vi "Main.vi"() -> ()   [LabVIEW 2009, in "Main.lvlib"]
doc: "Main robot program VI. Should be the start VI of the built program."
uses:
  Main.lvlib
  Drive/Drive_Point.ctl
  OWNCAN.lvlib
  NetworkVarTarget.lvlib
  MainVariables.lvlib
  Drive.lvlib
panel:
  in  "Goal point":T1
  out "error out":errorcluster
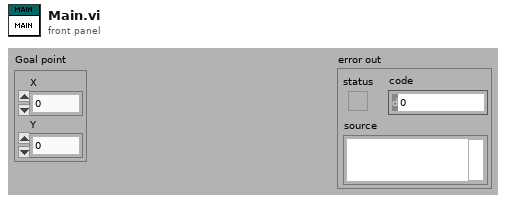
[diagram p1: front panel]
types:
  T1 = typedef "Drive.lvlib/Drive_Point.ctl" = cluster{"X":dbl, "Y":dbl}
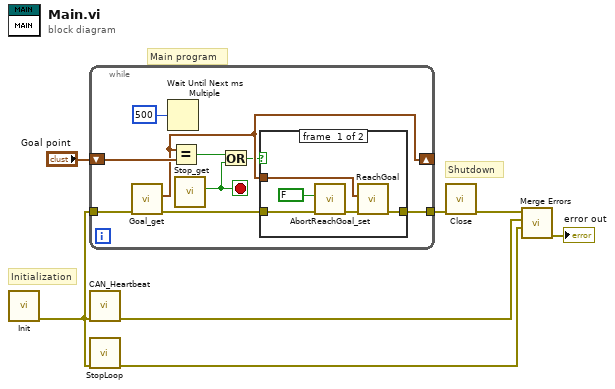
[diagram p0: block diagram]
diagram:
  # "Shutdown"
  # "Main program"
  # "Initialization"
  n1 = call "Init.vi"() -> ("error out"=w1:errorcluster)  [unwired: 11 in]
  n2 = while {
    tunnel: [w16] -> w7
    tunnel: w1 -> [w14]
    shift-right: [w11] -> _
    shift-left: "Goal point" -> [w15]
    stop <- w9 stop-if-true
    n3 = call "Goal_get.vi"("error in (no error)"=w14) -> ("error out"=w13:errorcluster, "Goal"=w11:cluster{"X":dbl, "Y":dbl})  [unwired: 9 in]
    n4 = Wait Until Next ms Multiple(millisecond multiple=u32 500) -> ()  [unwired: 1 out]
    n5 = Equal?(x=w11, y=w15) -> (x = y?=w8:bool)
    n6 = call "Stop_get.vi"() -> ("Stop"=w9:bool)  [unwired: 10 in, 1 out]
    n7 = Or(x=w8, y=w9) -> (x .or. y?=w10:bool)
    n8 = case shown="False" w10 {
      tunnel: [w21 w22] -> w16
      tunnel: w13 -> [w19 w22]
      tunnel: w11 -> [w18 _]
      frame #0 {
        n9 = call "AbortReachGoal_set.vi"("error in (no error)"=w19, "Abort? (F)"=FALSE) -> ("error out"=w20:errorcluster)  [unwired: 9 in]
        n10 = call "ReachGoal.vi"("error in"=w20, "Goal point"=w18) -> ("error out"=w21:errorcluster)  [unwired: 9 in]
      }
      frame #1 {
      }
    }
  }
  n11 = call "CAN_Heartbeat.vi"("error in"=w1) -> ("error out"=w4:errorcluster)  [unwired: 10 in]
  n12 = call "StopLoop.vi"("error in"=w1) -> ("error out"=w3:errorcluster)  [unwired: 10 in]
  n13 = call "Close.vi"("error in (no error)"=w7) -> ("error out"=w5:errorcluster)  [unwired: 10 in]
  n14 = call <vilib>:"Merge Errors.vi"("error in 3 (no error)"=w3, "error in 2 (no error)"=w4, "error in 1 (no error)"=w5) -> ("error out"=→"error out":errorcluster)  [unwired: 4 in]
